vi "Initialize DO Channel Settings.vi"(11 "array size":i32=8) -> (3 "channel settings":T1[](array[typedef]))   [LabVIEW 2017, in "Module Test.lvclass"]
uses:
  Module Test Classes/Module Test.lvclass
  Scripting/Modules/Mode Classes/Controls/digital channel settings.ctl
  Scripting/Scan Engine Scripting.lvlib
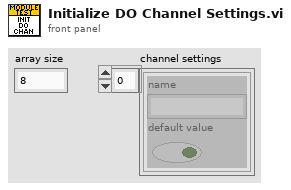
[diagram p1: front panel]
types:
  T1 = typedef "Scan Engine Scripting.lvlib/digital channel settings.ctl" = cluster{"name":string, "default value":bool}
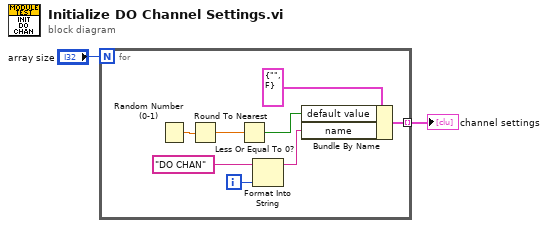
[diagram p0: block diagram]
diagram:
  n1 = for {
    N: "array size" -> [_]
    tunnel: [w6] -> w2 mode=indexing
    i -> [w5]
    n2 = Random Number (0-1)() -> (number: 0 to 1=w10:dbl)
    n3 = Round To Nearest(number=w10) -> (nearest integer value=w9:dbl)
    n4 = Less Or Equal To 0?(x=w9) -> (x <= 0?=w7:bool)
    n5 = Format Into String(initial string="DO CHAN", w5) -> (resulting string=w3:string)  [unwired: 2 in, 1 out]
    n6 = Bundle By Name(cluster=T1 {"name"="", "default value"=FALSE} ("channel settings"), "default value"=w7, "name"=w3) -> (w6:T1)
  }
  "channel settings" <- w2
